vi "Enqueue Handle Error.vi"(8 "error in":errorcluster) -> (0 "no error out":errorcluster, 5 "MHL Channel out":T1)   [LabVIEW 2025]
uses:
  <extravilib>/ChannelInstances/Event Messenger-c(str,var)/))Channel.ctl
  <extravilib>/ChannelInstances/Event Messenger-c(str,var)/))Channel.vi
  <extravilib>/ChannelInstances/Event Messenger-c(str,var).lvlib
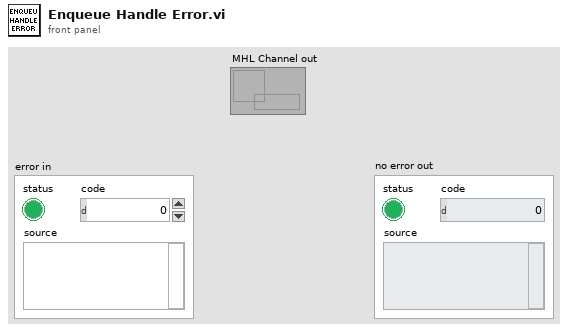
[diagram p1: front panel]
types:
  T1 = typedef "Event Messenger-c(str,var).lvlib/))Channel.ctl" = refnum<queue>
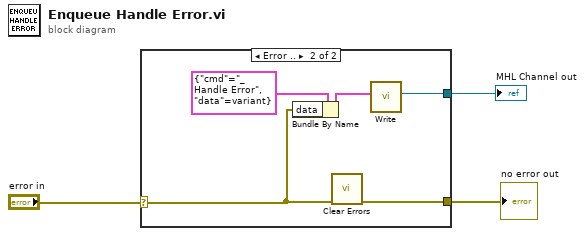
[diagram p0: block diagram]
diagram:
  n1 = case shown="Error .." "error in" {
    selector: "error in" -> [w4 w6]
    tunnel: [_ w9] -> w3
    tunnel: [w4 w5] -> w1
    frame No Error {
    }
    frame Error {
      n2 = Bundle By Name(cluster=cluster{"cmd":string, "data":variant} {"cmd"="_Handle Error", "data"=variant} ("element"), "data"=w6) -> (w7:cluster{"cmd":string, "data":variant})
      n3 = call <vilib>:"Clear Errors.vi"("error in (no error)"=w6) -> ("error out"=w5:errorcluster)  [unwired: 5 in, 1 out]
      n4 = call <extravilib>:"Write.vi"("element"=w7) -> ("channel"=w9:T1)  [unwired: 9 in, 1 out]
    }
  }
  "MHL Channel out" <- w3
  "no error out" <- w1
